vi "SD-image color table presets.vi"(11 "Color table":T1=enum."enhance low") -> (2 "Make new one cancelled":bool, 3 "white to yellow color table":u32[](array[numeric]))   [LabVIEW 2020]
uses:
  SD-image color table presets.ctl
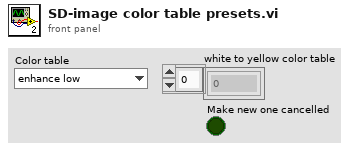
[diagram p1: front panel]
types:
  T1 = typedef "SD-image color table presets.ctl" = enum16{"Greyscale", "Binary", "Gradient", "Rainbow", "Temperature", "enhance low", "blue yellow red", "BYR enhance low", "white blue yellow", "BWR enhance low", "make a new one"}
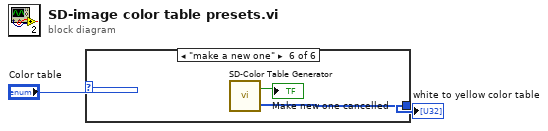
[diagram p0: block diagram]
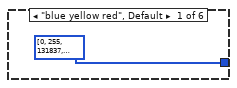
[diagram p2: hidden frame]
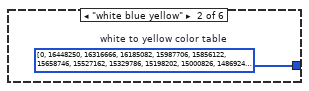
[diagram p3: hidden frame]
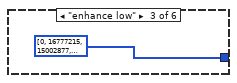
[diagram p4: hidden frame]
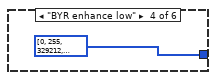
[diagram p5: hidden frame]
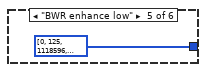
[diagram p6: hidden frame]
diagram:
  n1 = case shown="\"make a new one\"" "Color table" {
    tunnel: [u32[] [0, 255, 131837, 263419, 395001, 526583, 658165, 855284, 987122, 1118704, 1250286, 1381868, 1513450, 1645032, 1776614, 1908196, 2039778, 2171361, 2368479, 2500061, 2631643, 2763225, 2895063, 3026645, 3158227, 3289809, 3421391, 3552974, 3684556, 3881674, 4013256, 4144838, 4276420, 4408002, 4539584, 4671166, 4803004, 4934587, 5066169, 5197751, 5394869, 5526451, 5658033, 5789615, 5921197, 6052779, 6184361, 6315944, 6447526, 6579364, 6710946, 6908064, 7039646, 7171228, 7302810, 7434392, 7565974, 7697557, 7829139, 7960721, 8092303, 8223885, 8421003, 8552841, 8684423, 8816005, 8947587, 9079170, 9210752, 9342334, 9473916, 9605498, 9737080, 9868662, 10065780, 10197362, 10328944, 10460782, 10592365, 10723947, 10855529, 10987111, 11118693, 11250275, 11381857, 11578975, 11710557, 11842139, 11973722, 12105304, 12237142, 12368724, 12500306, 12631888, 12763470, 12895052, 13092170, 13223752, 13355335, 13486917, 13618499, 13750081, 13881663, 14013245, 14145083, 14276665, 14408247, 14605365, 14736948, 14868530, 15000112, 15131694, 15263276, 15394858, 15526440, 15658022, 15789604, 15921186, 16118561, 16250143, 16381725, 16513307, 16644889, 16776471, 16776981, 16776467, 16775953, 16775439, 16774926, 16774412, 16773898, 16773384, 16772870, 16772356, 16771844, 16771332, 16770820, 16770564, 16770052, 16769540, 16769028, 16768516, 16768004, 16767492, 16766980, 16766468, 16765956, 16765444, 16764932, 16764419, 16763907, 16763395, 16762883, 16762371, 16761859, 16761347, 16760835, 16760323, 16759811, 16759299, 16758787, 16758275, 16757763, 16757251, 16756995, 16756483, 16755971, 16755459, 16754947, 16754435, 16753923, 16753411, 16752899, 16752387, 16751875, 16751363, 16750851, 16750339, 16749827, 16749314, 16748802, 16748290, 16747778, 16747266, 16746754, 16746242, 16745730, 16745218, 16744706, 16744450, 16743938, 16743426, 16742914, 16742402, 16741890, 16741378, 16740866, 16740354, 16739842, 16739330, 16738818, 16738306, 16737794, 16737282, 16736770, 16736258, 16735746, 16735234, 16734722, 16734209, 16733697, 16733185, 16732673, 16732161, 16731649, 16731137, 16730881, 16730369, 16729857, 16729345, 16728833, 16728321, 16727809, 16727297, 16726785, 16726273, 16725761, 16725249, 16724737, 16724225, 16723713, 16723201, 16722689, 16722177, 16721665, 16721153, 16720641, 16720129, 16719617, 16719104, 16718592, 16718336, 16717824, 16717312, 16716800, 16716288, 16715776, 16715264, 16714752, 16714240, 16713728, 16713216, 16712704, 16712192, 16711680, 16711680] ("blue yellow red Color Table") w4 u32[] [0, 16777215, 15002877, 13228283, 11453945, 9745143, 7970549, 6196211, 4421617, 2647279, 2707949, 2768363, 2829033, 2894567, 2894565, 2959843, 3025377, 3090911, 3156445, 3221979, 3287513, 3352790, 3352788, 3418322, 3483856, 3549390, 3614924, 3680202, 3745736, 3811270, 3811268, 3876802, 3942336, 4007614, 4073148, 4138682, 4204216, 4269750, 4269492, 4335026, 4400560, 4466095, 4531630, 4597166, 4662445, 4727980, 4727979, 4793514, 4859049, 4924585, 4989864, 5055399, 5120934, 5186469, 5186468, 5252004, 5317283, 5382818, 5448353, 5513888, 5579424, 5644703, 5710238, 5710237, 5775772, 5841307, 5906843, 5972122, 6037657, 6103192, 6168727, 6168727, 6234262, 6299541, 6365076, 6430611, 6496146, 6561682, 6627217, 6626960, 6692495, 6758030, 6823565, 6889101, 6954636, 7019915, 7085450, 7085449, 7150985, 7216520, 7281799, 7347334, 7412869, 7478404, 7543940, 7543939, 7609218, 7674753, 7740288, 7805823, 7871359, 7936894, 8002173, 8002172, 8067707, 8133243, 8198778, 8264313, 8329592, 8395127, 8460662, 8526198, 8526197, 8591476, 8657011, 8722546, 8788081, 8853617, 8919152, 8984431, 8984430, 9049965, 9115501, 9181036, 9246571, 9311850, 9377385, 9442920, 9442920, 9508455, 9573990, 9639269, 9704804, 9770340, 9835875, 9901410, 9901153, 9966688, 10032223, 10097759, 10163294, 10228829, 10294108, 10359643, 10359642, 10425178, 10490713, 10556248, 10621527, 10687062, 10752598, 10818133, 10818132, 10883667, 10948946, 11014481, 11080017, 11145552, 11211087, 11276366, 11341901, 11341900, 11407436, 11472971, 11538506, 11603785, 11669320, 11734856, 11800391, 11800390, 11865925, 11931204, 11996739, 12062275, 12127810, 12193345, 12258880, 12258623, 12324159, 12389694, 12455229, 12520764, 12586043, 12651578, 12717114, 12717113, 12782648, 12848183, 12913462, 12978997, 13044533, 13110068, 13175603, 13175602, 13240881, 13306417, 13371952, 13437487, 13503022, 13568557, 13633836, 13633836, 13699371, 13764906, 13830441, 13895976, 13961255, 14026791, 14092326, 14157861, 14157860, 14223139, 14288675, 14354210, 14419745, 14485280, 14550815, 14616094, 14616094, 14681629, 14747164, 14812699, 14878234, 14943513, 15009049, 15074584, 15074583, 15140118, 15205653, 15270933, 15336468, 15402003, 15467538, 15533073, 15532816, 15598352, 15663887, 15729422, 15794957, 15860492, 15925772, 15991307, 15991306, 16056841, 16122376, 16187911, 16253191, 16318726, 16384261, 16449796, 16449795, 16515330, 16580610, 16646145, 16711680, 16711680] u32[] [0, 255, 329212, 658168, 987381, 1316337, 1645294, 1974250, 2303207, 2632419, 2961376, 3290332, 3619289, 3948245, 4277458, 4606414, 4935371, 5264328, 5593284, 5922497, 6251453, 6580410, 6909366, 7238323, 7567535, 7896492, 8225448, 8554405, 8883617, 9212574, 9541530, 9870487, 10199443, 10528656, 10857613, 11186569, 11515526, 11844482, 12173695, 12502651, 12831608, 13160564, 13489521, 13818733, 14147690, 14476646, 14805603, 15134559, 15463772, 15792729, 16121685, 16449106, 16776526, 16776011, 16775751, 16775492, 16775232, 16774717, 16774457, 16774198, 16773938, 16773423, 16773163, 16772904, 16772648, 16772136, 16771879, 16771623, 16771367, 16770855, 16770599, 16770342, 16770086, 16769574, 16769318, 16769061, 16768805, 16768293, 16768037, 16767781, 16767524, 16767012, 16766756, 16766500, 16766244, 16765731, 16765475, 16765219, 16764963, 16764451, 16764194, 16763938, 16763682, 16763170, 16762914, 16762657, 16762401, 16761889, 16761633, 16761376, 16761120, 16760608, 16760352, 16760096, 16759839, 16759327, 16759071, 16758815, 16758559, 16758046, 16757790, 16757534, 16757278, 16756766, 16756509, 16756253, 16755997, 16755485, 16755228, 16754972, 16754716, 16754204, 16753948, 16753691, 16753435, 16752923, 16752667, 16752411, 16752154, 16751642, 16751386, 16751130, 16750874, 16750361, 16750105, 16749849, 16749593, 16749081, 16748824, 16748568, 16748312, 16747800, 16747543, 16747287, 16747031, 16746519, 16746263, 16746006, 16745750, 16745238, 16744982, 16744726, 16744469, 16743957, 16743701, 16743445, 16743189, 16742676, 16742420, 16742164, 16741908, 16741395, 16741139, 16740883, 16740627, 16740115, 16739858, 16739602, 16739346, 16738834, 16738578, 16738321, 16738065, 16737553, 16737297, 16737041, 16736784, 16736272, 16736016, 16735760, 16735503, 16734991, 16734735, 16734479, 16734223, 16733710, 16733454, 16733198, 16732942, 16732430, 16732173, 16731917, 16731661, 16731149, 16730893, 16730636, 16730380, 16729868, 16729612, 16729356, 16729099, 16728587, 16728331, 16728075, 16727818, 16727306, 16727050, 16726794, 16726538, 16726025, 16725769, 16725513, 16725257, 16724745, 16724488, 16724232, 16723976, 16723464, 16723208, 16722951, 16722695, 16722183, 16721927, 16721670, 16721414, 16720902, 16720646, 16720390, 16720133, 16719621, 16719365, 16719109, 16718853, 16718340, 16718084, 16717828, 16717572, 16717060, 16716803, 16716547, 16716291, 16715779, 16715523, 16715266, 16715010, 16714498, 16714242, 16713985, 16713729, 16713217, 16712961, 16712705, 16712448, 16711936, 16711680, 16711680] ("Array") u32[] [0, 125, 1118596, 2237066, 3355537, 4474008, 5592479, 6710949, 7829420, 8947891, 10066362, 11184832, 12303303, 13421774, 14540245, 15658715, 16777186, 16776937, 16776688, 16776438, 16776189, 16775932, 16775675, 16775162, 16774905, 16774648, 16774391, 16774133, 16773876, 16773619, 16773362, 16773105, 16772848, 16772591, 16772334, 16772077, 16771820, 16771307, 16771050, 16770792, 16770535, 16770278, 16770021, 16769764, 16769507, 16769250, 16768993, 16768736, 16768479, 16768222, 16767965, 16767451, 16767194, 16766937, 16766680, 16766423, 16766166, 16765909, 16765652, 16765395, 16765138, 16764881, 16764624, 16764367, 16764109, 16763596, 16763339, 16763082, 16762825, 16762568, 16762311, 16762054, 16761797, 16761540, 16761283, 16761026, 16760768, 16760511, 16760254, 16759741, 16759484, 16759227, 16758970, 16758713, 16758456, 16758199, 16757942, 16757685, 16757427, 16757170, 16756913, 16756656, 16756399, 16755886, 16755629, 16755372, 16755115, 16754858, 16754601, 16754344, 16754087, 16753829, 16753572, 16753315, 16753058, 16752801, 16752544, 16752031, 16751774, 16751517, 16751260, 16751003, 16750746, 16750488, 16750231, 16749974, 16749717, 16749460, 16749203, 16748946, 16748689, 16748176, 16747919, 16747662, 16747405, 16747147, 16746890, 16746633, 16746376, 16746119, 16745862, 16745605, 16745348, 16745091, 16744834, 16744321, 16744064, 16743806, 16743549, 16743292, 16743035, 16742778, 16742521, 16742264, 16742007, 16741750, 16741493, 16741236, 16740979, 16740466, 16740208, 16739951, 16739694, 16739437, 16739180, 16738923, 16738666, 16738409, 16738152, 16737895, 16737638, 16737381, 16737123, 16736610, 16736353, 16736096, 16735839, 16735582, 16735325, 16735068, 16734811, 16734554, 16734297, 16734040, 16733782, 16733525, 16733268, 16732755, 16732498, 16732241, 16731984, 16731727, 16731470, 16731213, 16730956, 16730699, 16730442, 16730184, 16729927, 16729670, 16729413, 16728900, 16728643, 16728386, 16728129, 16727872, 16727615, 16727358, 16727101, 16726843, 16726586, 16726329, 16726072, 16725815, 16725558, 16725045, 16724788, 16724531, 16724274, 16724017, 16723760, 16723502, 16723245, 16722988, 16722731, 16722474, 16722217, 16721960, 16721703, 16721190, 16720933, 16720676, 16720419, 16720162, 16719904, 16719647, 16719390, 16719133, 16718876, 16718619, 16718362, 16718105, 16717848, 16717335, 16717078, 16716821, 16716563, 16716306, 16716049, 16715792, 16715535, 16715278, 16715021, 16714764, 16714507, 16714250, 16713993, 16713480, 16713222, 16712965, 16712708, 16712451, 16712194, 16711937, 16711680, 16711680] ("final for BELLA PRL") w9] -> w2
    frame "blue yellow red", Default {
    }
    frame "white blue yellow" {
      w4 = u32[] [0, 16448250, 16316666, 16185082, 15987706, 15856122, 15658746, 15527162, 15329786, 15198202, 15000826, 14869242, 14737658, 14540282, 14408698, 14211322, 14079738, 13882362, 13750778, 13553402, 13421818, 13224442, 13092859, 12961275, 12763899, 12632315, 12434939, 12303355, 12105979, 11974395, 11777019, 11645435, 11448059, 11316475, 11184891, 10987515, 10855931, 10658555, 10526971, 10329595, 10198011, 10000635, 9869052, 9737468, 9540092, 9408508, 9211132, 9079548, 8882172, 8750588, 8553212, 8421628, 8224252, 8092668, 7961084, 7763708, 7632124, 7434748, 7303164, 7105788, 6974204, 6776828, 6645244, 6447869, 6316285, 6184701, 5987325, 5855741, 5658365, 5526781, 5329405, 5197821, 5000445, 4868861, 4737277, 4539901, 4408317, 4210941, 4079357, 3881981, 3750397, 3553021, 3421437, 3224062, 3092478, 2960894, 2763518, 2631934, 2434558, 2302974, 2105598, 1974014, 1776638, 1645054, 1447678, 1316094, 1184510, 987134, 855550, 658174, 526590, 329214, 197630, 254, 131324, 327930, 524535, 721141, 918003, 1114608, 1311214, 1507820, 1638889, 1835751, 2032356, 2228962, 2425568, 2622173, 2819035, 2950105, 3146710, 3343316, 3539922, 3736783, 3933389, 4129995, 4261064, 4457670, 4654531, 4851137, 5047743, 5244348, 5440954, 5637816, 5768885, 5965491, 6162097, 6358702, 6555564, 6752169, 6948775, 7079845, 7276450, 7473312, 7669918, 7866523, 8063129, 8259735, 8456596, 8587666, 8784272, 8980877, 9177483, 9374344, 9570950, 9767556, 9898625, 10095231, 10292093, 10488698, 10685304, 10881910, 11078515, 11275377, 11406446, 11603052, 11799658, 11996263, 12193125, 12389731, 12586336, 12717406, 12914012, 13110873, 13307479, 13504085, 13700690, 13897296, 14028621, 14225227, 14421833, 14618438, 14815044, 15011906, 15208511, 15405117, 15536187, 15732792, 15929654, 16126259, 16322865, 16519471, 16716332, 16717356, 16718380, 16719404, 16720428, 16721708, 16722732, 16723756, 16724780, 16725804, 16727084, 16728108, 16729132, 16730156, 16731180, 16732204, 16733484, 16734508, 16735532, 16736555, 16737579, 16738859, 16739883, 16740907, 16741931, 16742955, 16744235, 16745259, 16746283, 16747307, 16748331, 16749611, 16750635, 16751659, 16752683, 16753707, 16754731, 16756011, 16757034, 16758058, 16759082, 16760106, 16761386, 16762410, 16763434, 16764458, 16765482, 16766762, 16767786, 16768810, 16769834, 16770858, 16771882, 16773162, 16774186, 16775210, 16775989, 16776018, 16776303, 16776332, 16776616, 16776645, 16448250, 2027264]  # white to yellow color table
    }
    frame "enhance low" {
    }
    frame "BYR enhance low" {
    }
    frame "BWR enhance low" {
    }
    frame "make a new one" {
      n2 = call "SD-Color Table Generator.vi"() -> (0:w9:u32[], "Cancel 2"=→"Make new one cancelled":bool)  [unwired: 2 in]
    }
  }
  "white to yellow color table" <- w2
